vi "Init with SQL Records.vi"(8 "error in (no error)":errorcluster, 10 "SQL Dataset":variant[][](array[variant]), 11 "Credit Statement in":refnum<class "Credit Statement.lvclass">) -> (0 "error out":errorcluster, 3 "Credit Statement out":refnum<class "Credit Statement.lvclass">)   [LabVIEW 2018, in "Credit Statement.lvclass"]
uses:
  Credit Statement.lvclass
  Credit Record/Credit Transaction.lvclass
  Credit Statement.lvclass/Credit Statement.ctl
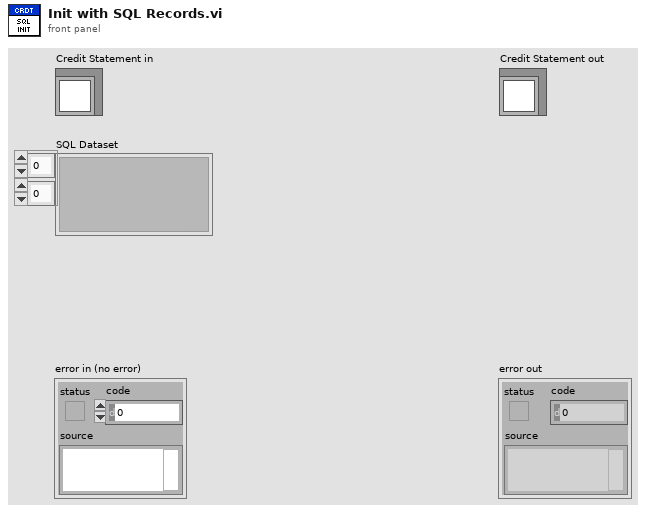
[diagram p1: front panel]
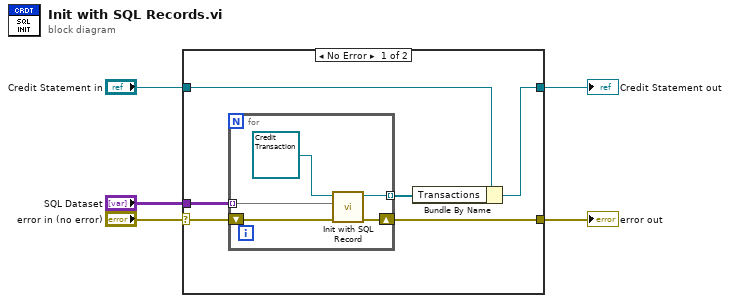
[diagram p0: block diagram]
diagram:
  n1 = case shown="No Error" "error in (no error)" {
    selector: "error in (no error)" -> [w11 w18]
    tunnel: "Credit Statement in" -> [w8 w17]
    tunnel: "SQL Dataset" -> [w10 _]
    tunnel: [w9 w18] -> w1
    tunnel: [w7 w17] -> w2
    frame No Error {
      n2 = for {
        shift-right: [w15] -> w9
        shift-left: w11 -> [w16]
        tunnel: w10 -> [w13] mode=indexing
        tunnel: [w14] -> w6 mode=indexing
        n3 = call-dynamic "Init with SQL Record.vi"("error in (no error)"=w16, "MySQL Record"=w13, "Credit Transaction in"=refnum<class "Credit Transaction.lvclass"> refnum ("Credit Transaction.lvclass")) -> ("error out"=w15:errorcluster, "Credit Transaction out"=w14:refnum<class "Credit Transaction.lvclass">)  [unwired: 7 in]
      }
      n4 = Bundle By Name(cluster=w8, "Transactions"=w6) -> (w7:refnum<class "Credit Statement.lvclass">)
    }
    frame Error {
    }
  }
  "error out" <- w1
  "Credit Statement out" <- w2
